vi "AMB_Create_CAN_ID.vi"(1 "Relative Address in":u32 format="%.0x", 2 "Slave Node in":cluster{"Address":i16, "Serial Number":i8[]} {"Serial Number" format="%.0x"; "Address" format="%.0x"}) -> (0 "CAN ID out":u32 format="%.0x")   [LabVIEW 2017]
doc: "AMB Create CAN ID\nCreate a CAN message ID from a slave node cluster\nand a relative address. Also sets flag for 29 bit addressing."
panel:
  # "ALMA Monitor and Control Bus\nCreate CAN ID"
  # "Node Address"
  # "Serial Number"
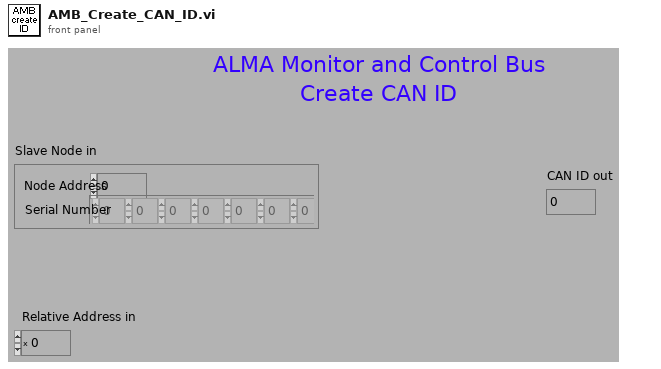
[diagram p1: front panel]
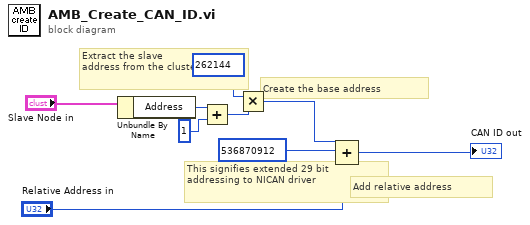
[diagram p0: block diagram]
diagram:
  # "This signifies extended 29 bit\naddressing to NICAN driver"
  # "Add relative address"
  # "Create the base address"
  # "Extract the slave\naddress from the cluster"
  n1 = Unbundle By Name("Slave Node in") -> ("Address"=w7:i16)
  n2 = Add(x=w7, y=i8 1) -> (x+y=w5:i16)
  n3 = Multiply(x=u32 262144, y=w5) -> (x*y=w8:u32)
  n4 = Compound Arithmetic op=ADD(w8, u32 536870912, "Relative Address in") -> (→"CAN ID out":u32)
